vi "Listen to RPi.vi"(8 "error in (no error)":errorcluster, 9 "port":u16, 10 "service name":string, 11 "net address":u32) -> (0 "error out":errorcluster)   [LabVIEW 2016, in "Huskie Swerve.lvlib"]
uses:
  Huskie Swerve.lvlib
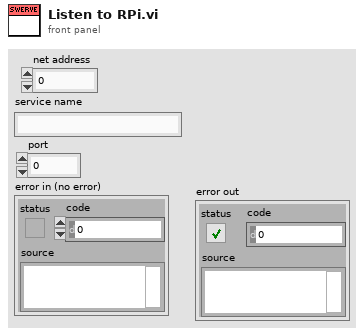
[diagram p1: front panel]
types:
  T1 = enum16{"Standard", "Buffered", "CRLF", "Immediate"}
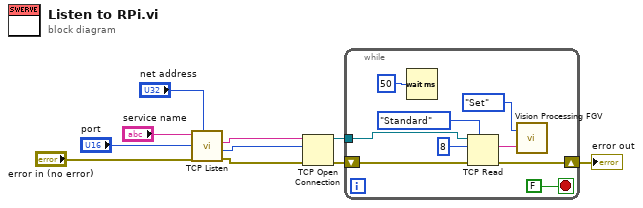
[diagram p0: block diagram]
diagram:
  n1 = call <vilib>:"TCP Listen.vi"("net address"="net address", "error in (no error)"="error in (no error)", "port"="port", "service name"="service name") -> ("error out"=w7:errorcluster, "remote port"=w6:u16, "remote address"=w8:string)  [unwired: 3 in, 2 out]
  n2 = TCP Open Connection(address=w8, remote port or service name=w6, error in (no error)=w7) -> (connection ID=w10:refnum<k5>, error out=w9:errorcluster)  [unwired: 2 in]
  n3 = while {
    tunnel: w10 -> [w15]
    shift-right: [w18] -> w1
    shift-left: w9 -> [w19]
    stop <- FALSE stop-if-true
    n4 = Wait (ms)(milliseconds to wait=u32 50) -> ()  [unwired: 1 out]
    n5 = TCP Read(connection ID=w15, bytes to read=8, error in (no error)=w19, 7:T1."Standard" ("mode (standard)")) -> (data out=w17:string, error out=w18:errorcluster)  [unwired: 1 in, 1 out]
    n6 = call "Vision Processing FGV.vi"("New Vision Processing"=w17, "Action"=enum16{"Set", "Get"}."Set") -> ()  [unwired: 1 out]
  }
  "error out" <- w1
